vi "oa_Perform Vector Averaging (1 Channel).vi"(6 "averaging state info in":T1 {"averages completed" format="%.2f"; "power spectrum" min=0.0 max=127.0 format="%.2f"; "complex FFT" format="%.2f"}, 7 "processing control in":T2(ring), 8 "error in (no error)":errorcluster, 9 "averaging parameters":T3={"averaging mode"=enum."No averaging", "weighting mode"=enum."Exponential", "number of averages"=10, "linear mode"=enum."One shot"} {"number of averages" min=1 step=1}, 10 "spectrum settings":cluster{"window type":u32, "block size":i32}={"window type"=1, "block size"=400} {"block size" min=2; "window type" items=["None"=0, "Hanning"=1, "Hamming"=2, "Blackman-Harris"=3, "Exact Blackman"=4, "Blackman"=5, "Flat Top"=6, "4 Term B-Harris"=7, "7 Term B-Harris"=8, "Low Sidelobe"=9, "Gaussian"=62]}, 11 "Y":cdb[][](array[numeric]) format="%.2f") -> (0 "error out":errorcluster, 1 "averages completed":dbl, 2 "averaging done":bool, 3 "Y out":cdb[](array[numeric]) format="%.2f", 4 "averaging state info out":T1 {"averages completed" format="%.2f"; "power spectrum" min=0.0 max=127.0 format="%.2f"; "complex FFT" format="%.2f"})   [LabVIEW 2017, in "SoundVib_Resampling.lvlib"]
uses:
  <vilib>/addons/Sound and Vibration/Order Analysis/Resample Order Tracking/SoundVib_Resampling.lvlib
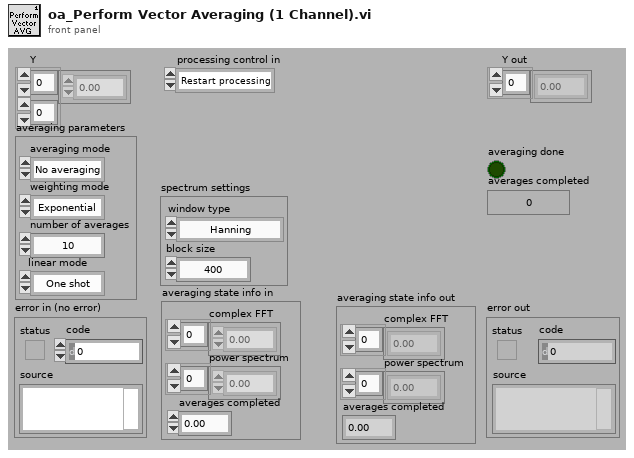
[diagram p1: front panel]
types:
  T1 = cluster{"complex FFT":cdb[], "power spectrum":dbl[], "averages completed":dbl}
  T2 = enum16{"Restart processing", "Continue processing", "Skip processing"}
  T3 = cluster{"averaging mode":enum16{"No averaging", "Vector averaging", "RMS averaging", "Peak hold"}, "weighting mode":enum16{"Linear", "Exponential"}, "number of averages":u32, "linear mode":enum16{"One shot", "Auto restart"}}
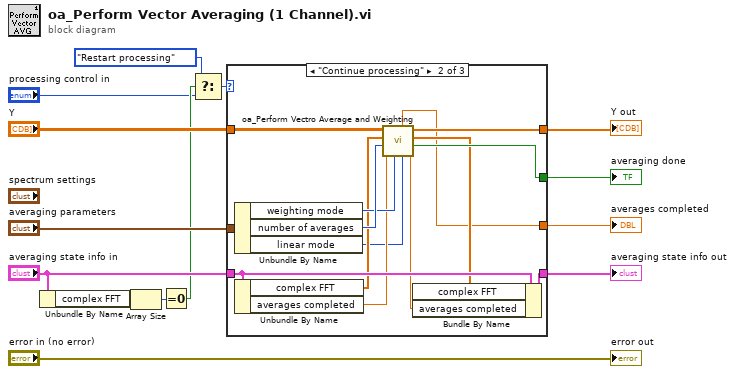
[diagram p0: block diagram]
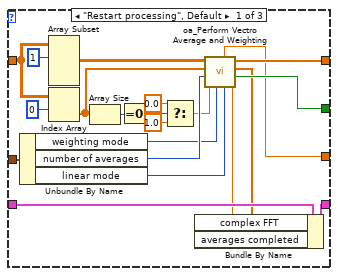
[diagram p2: hidden frame]
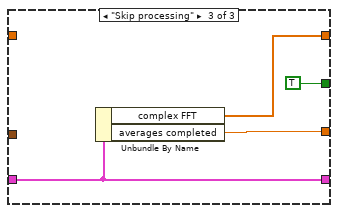
[diagram p3: hidden frame]
diagram:
  n1 = Unbundle By Name("averaging state info in") -> ("complex FFT"=w7:cdb[])
  n2 = Array Size(array=w7) -> (size(s)=w6:i32)
  n3 = Equal To 0?(x=w6) -> (x = 0?=w5:bool)
  n4 = Select(t=T2."Restart processing", s=w5, f="processing control in") -> (s? t:f=w4:T2)
  n5 = case shown="\"Continue processing\"" w4 {
    tunnel: "averaging parameters" -> [w33 w43 _]
    tunnel: "Y" -> [w26 w40 _]
    tunnel: "averaging state info in" -> [w35 w45 w52]
    tunnel: [w34 w46 w52] -> w12
    tunnel: [w15 w37 w51] -> w11
    tunnel: [w31 w47 TRUE] -> w10
    tunnel: [w29 w42 w50] -> w1
    frame "Restart processing", Default {
      n6 = Unbundle By Name(w33) -> ("weighting mode"=w30:enum16{"Linear", "Exponential"}, "number of averages"=w32:u32, "linear mode"=w17:enum16{"One shot", "Auto restart"})
      n7 = Array Subset(array=w26, index (row)=1 ("index")) -> (w25:cdb[][])  [unwired: 3 in]
      n8 = Index Array(array=w26, index (row)=0) -> (element=w23:cdb[])  [unwired: 1 in]
      n9 = Array Size(array=w23) -> (size(s)=w24:i32)
      n10 = Equal To 0?(x=w24) -> (x = 0?=w22:bool)
      n11 = Select(t=0.0, s=w22, f=1.0) -> (s? t:f=w18:dbl)
      n12 = call <vilib>:"oa_Perform Vectro Average and Weighting.vi"("linear mode"=w17, "weighting mode"=w30, "averages completed"=w18, "number of averages"=w32, "previous array"=w23, "Y"=w25) -> ("averages completed for buffer"=w19:dbl, "average done?"=w31:bool, "complex spectrum for buffer"=w16:cdb[], "complex spectrum output"=w29:cdb[], "averages completed for output"=w15:dbl)  [unwired: 1 in]
      n13 = Bundle By Name(cluster=w35, "complex FFT"=w16, "averages completed"=w19) -> (w34:T1)
    }
    frame "Continue processing" {
      n14 = Unbundle By Name(w43) -> ("weighting mode"=w48:enum16{"Linear", "Exponential"}, "number of averages"=w49:u32, "linear mode"=w39:enum16{"One shot", "Auto restart"})
      n15 = Unbundle By Name(w45) -> ("complex FFT"=w44:cdb[], "averages completed"=w41:dbl)
      n16 = call <vilib>:"oa_Perform Vectro Average and Weighting.vi"("linear mode"=w39, "weighting mode"=w48, "averages completed"=w41, "number of averages"=w49, "previous array"=w44, "Y"=w40) -> ("averages completed for buffer"=w36:dbl, "average done?"=w47:bool, "complex spectrum for buffer"=w38:cdb[], "complex spectrum output"=w42:cdb[], "averages completed for output"=w37:dbl)  [unwired: 1 in]
      n17 = Bundle By Name(cluster=w45, "complex FFT"=w38, "averages completed"=w36) -> (w46:T1)
    }
    frame "Skip processing" {
      n18 = Unbundle By Name(w52) -> ("complex FFT"=w50:cdb[], "averages completed"=w51:dbl)
    }
  }
  "averaging done" <- w10
  "averages completed" <- w11
  "Y out" <- w1
  "averaging state info out" <- w12
  "error out" <- "error in (no error)"
